vi "Binking.vi"() -> (0 "led2":bool, 1 "led1":bool)   [LabVIEW 2013]
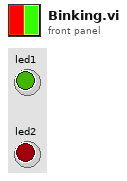
[diagram p1: front panel]
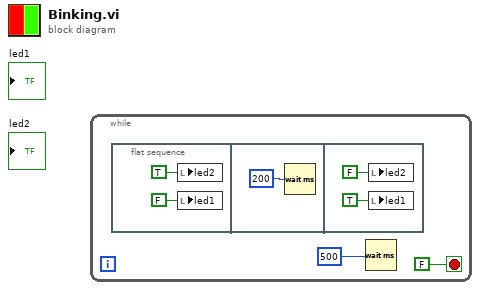
[diagram p0: block diagram]
diagram:
  n1 = while {
    stop <- FALSE stop-if-true
    n2 = flat-sequence {
      frame #0 {
        n3 = local write "led2"(TRUE ("led2")) -> ()
        n4 = local write "led1"(FALSE ("led1")) -> ()
      }
      frame #1 {
        n5 = Wait (ms)(milliseconds to wait=u32 200 ("millisecond timer value")) -> ()  [unwired: 1 out]
      }
      frame #2 {
        n6 = local write "led2"(FALSE ("led2")) -> ()
        n7 = local write "led1"(TRUE ("led1")) -> ()
      }
    }
    n8 = Wait (ms)(milliseconds to wait=u32 500 ("millisecond timer value")) -> ()  [unwired: 1 out]
  }
